vi "GreyRings.vi"(8 "error in (no error)":errorcluster, 11 "Maui Manager in":refnum<class "Maui Manager.lvclass">) -> (0 "error out":errorcluster, 3 "Maui Manager out":refnum<class "Maui Manager.lvclass">)   [LabVIEW 2020, in "Maui Manager.lvclass"]
uses:
  Maui Manager.lvclass
  Maui Manager.lvclass/Maui Manager.ctl
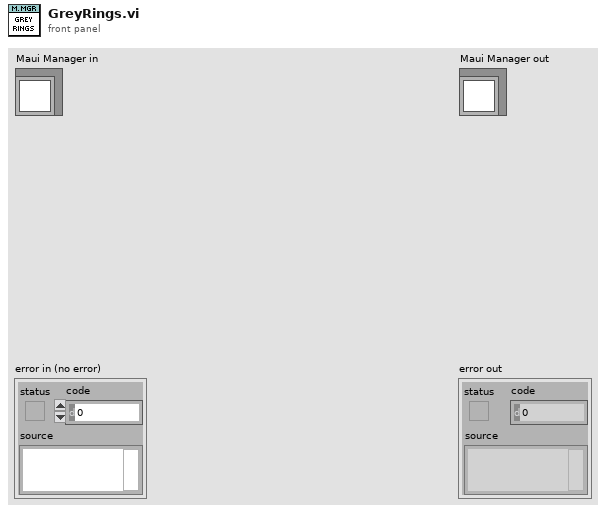
[diagram p1: front panel]
types:
  T1 = cluster{"Control":refnum<vi>, "Subpanel":refnum<vi>, "Active":i32, "Ctrl Class":string}[]
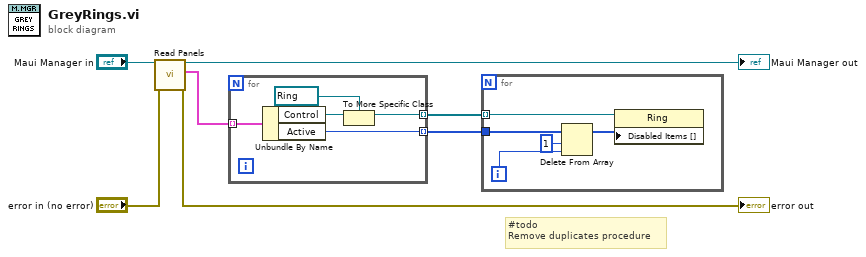
[diagram p0: block diagram]
diagram:
  # "#todo \nRemove duplicates procedure"
  n1 = call "Read Panels.vi"("error in (no error)"="error in (no error)", "Maui Manager in"="Maui Manager in") -> ("error out"=→"error out":errorcluster, "Panels"=w5:T1, "Maui Manager out"=→"Maui Manager out":refnum<class "Maui Manager.lvclass">)  [unwired: 7 in]
  n2 = for {
    tunnel: w5 -> [w12] mode=indexing
    tunnel: [w9] -> w4 mode=indexing
    tunnel: [w8] -> w3 mode=indexing
    n3 = Unbundle By Name(w12) -> ("Control"=w11:refnum<vi>, "Active"=w8:i32)
    n4 = To More Specific Class(target class=refnum<vi> refnum ("reference"), reference=w11) -> (specific class reference=w9:refnum<vi>)  [unwired: 1 in, 1 out]
  }
  n5 = for {
    tunnel: w4 -> [w14] mode=indexing
    tunnel: w3 -> [w17]
    i -> [w16]
    n6 = Delete From Array(array=w17, length=1, index=w16) -> (array with subset deleted=w13:i32[])  [unwired: 1 out]
    n7 = property class="Ring"(reference=w14, "Disabled Items []"=w13) -> ()  [unwired: 1 in, 2 out]
  }
